vi "Configuration Tool Main.vi"() -> ()   [LabVIEW 2013, in "Advanced Configuration Tool.lvlib"]
doc: "This is the main VI for the configuration editor."
uses:
  Advanced Configuration Tool.lvlib
  Controls/StateCluster.ctl
  CEF_TreeControl/Repository/NISE_CEF_Repository.lvclass
  CEF_TreeControl/Node/NodeRef.ctl
  CEF_TreeControl/Node/NISE_CEF_Node.lvclass
  CEF_TreeControl/Node/UserEventRef.ctl
  CEF_TreeControl/Controls/EventCluster.ctl
  Controls/AddMessage.ctl
  Controls/MoveMessage.ctl
  <vilib>/Utility/error.llb/DialogType.ctl
  Classes/cRIO node/cRIO  node root.lvclass
  CEF_TreeControl/hierarchy repo/NISE_CEF_HierarchyRepo.lvclass
  <vilib>/NI/AMC/Read Termination Message.vi
  <vilib>/NI/AMC/Create Single Message.vi
  <vilib>/NI/AMC/Update Message Routing Info.vi
  <vilib>/NI/AMC/Send Message.vi
  <vilib>/NI/AMC/Globals.vi
  <vilib>/NI/AMC/AMC.lvlib
  CEF_TreeControl/NISE_CEF_TreeControl.lvlib
panel:
  in  "View":string(tree)
  in  "Exit":bool
  # "Configurator"
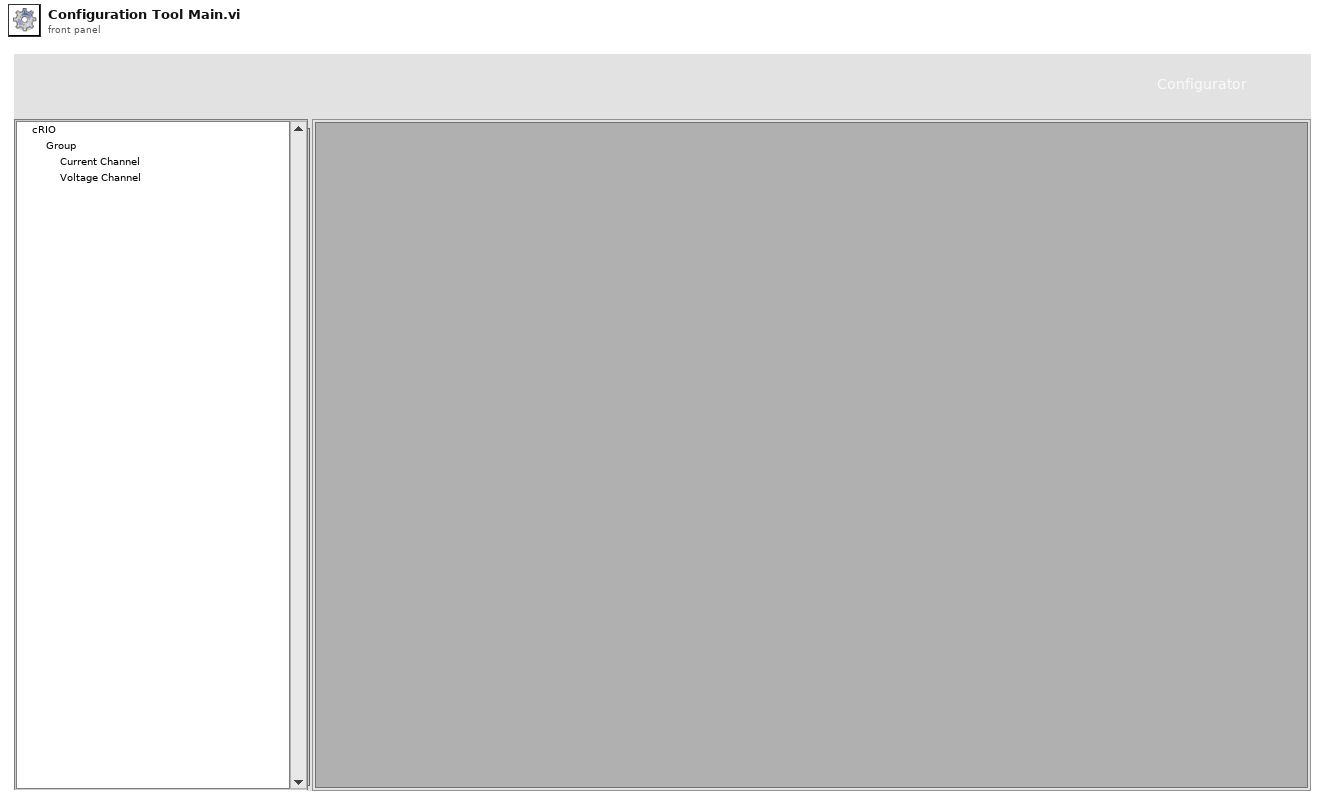
[diagram p1: front panel]
types:
  T1 = typedef "Advanced Configuration Tool.lvlib/StateCluster.ctl" = cluster{"repository":refnum<class "NISE_CEF_Repository.lvclass">, "root":T2, "unsaved changes":bool, "current path":path, "user event ref":T3, "glyph path":path, "classes path":path}
  T2 = typedef "NISE_CEF_Node.lvclass/NodeRef.ctl" = refnum<data-value>
  T3 = typedef "NISE_CEF_Node.lvclass/UserEventRef.ctl" = refnum<user-event>
  T4 = typedef "AMC.lvlib/Message Queue.ctl" = refnum<queue>
  T5 = typedef "Advanced Configuration Tool.lvlib/AddMessage.ctl" = cluster{"node type":string, "to add to":string}
  T6 = typedef "Advanced Configuration Tool.lvlib/MoveMessage.ctl" = cluster{"node ref":T2, "new parent":T2}
  T7 = typedef "NISE_CEF_TreeControl.lvlib/EventCluster.ctl" = cluster{"command":string, "data":string}
  T8 = typedef "Advanced Configuration Tool.lvlib/FilePaths.ctl" = cluster{"glyphs":path, "classes":path}
  T9 = typedef "DialogType.ctl" = u16
  T10 = typedef "NISE_CEF_Node.lvclass/Summary.ctl" = cluster{"ID":string, "parent ID":string, "node type":string, "text":string, "additional text":string, "glyph":string, "depth":i32}
  T11 = typedef "LVPoint32TypeDef.ctl" = cluster{"Horizontal":i32, "Vertical":i32}
  T12 = cluster{"data name":string, "drag data":variant}[]
  T13 = typedef "NISE_CEF_Node.lvclass/NodeMenuOptions.ctl" = cluster{"removable":bool, "movable":bool, "duplicate":bool}
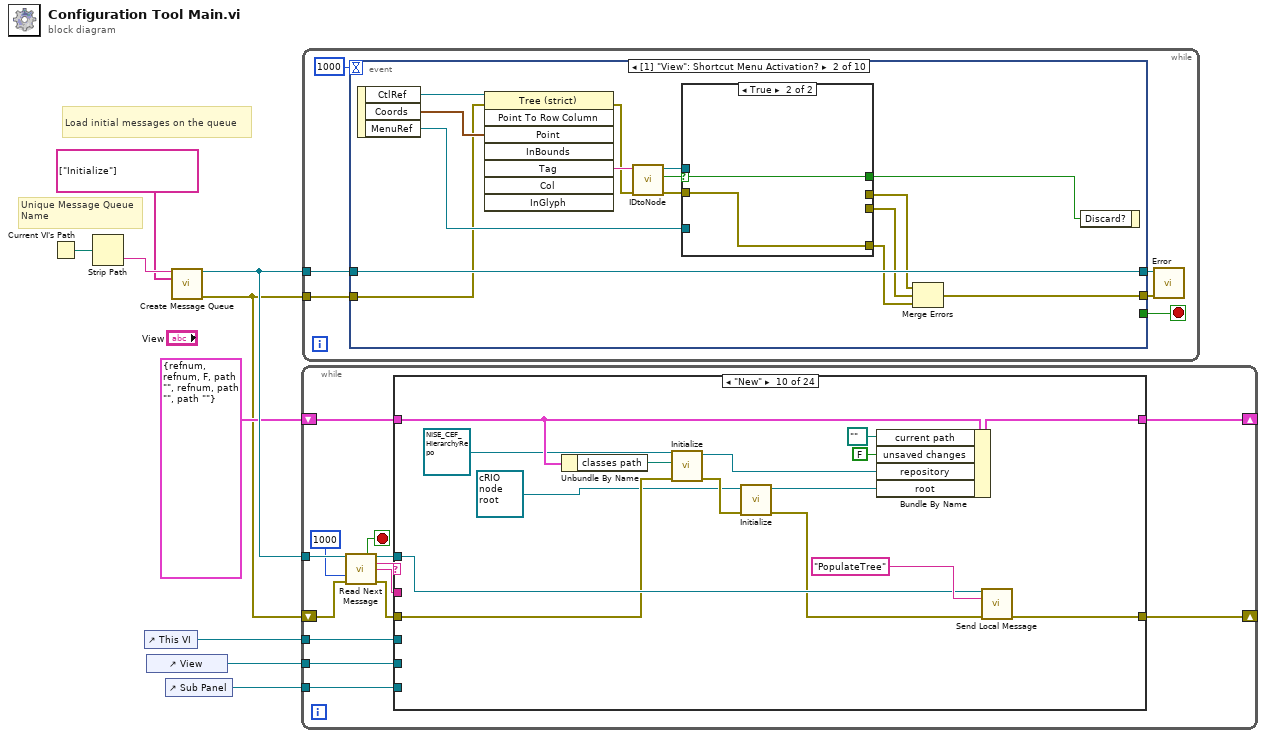
[diagram p0: block diagram]
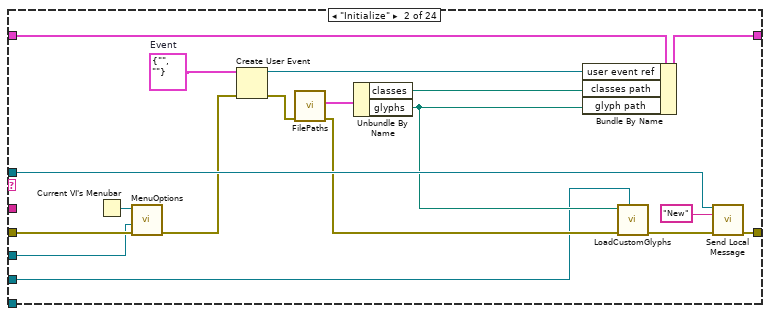
[diagram p3: hidden frame]
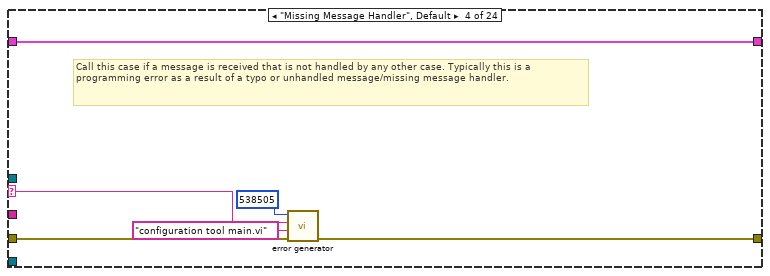
[diagram p5: hidden frame]
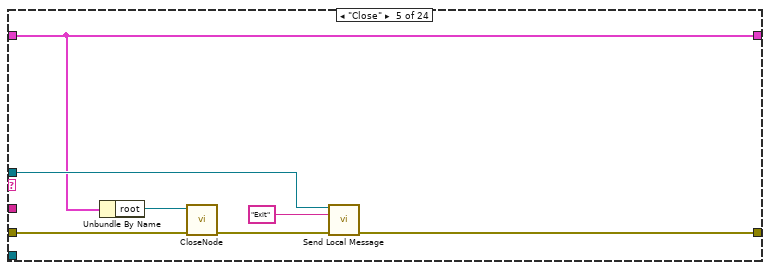
[diagram p6: hidden frame]
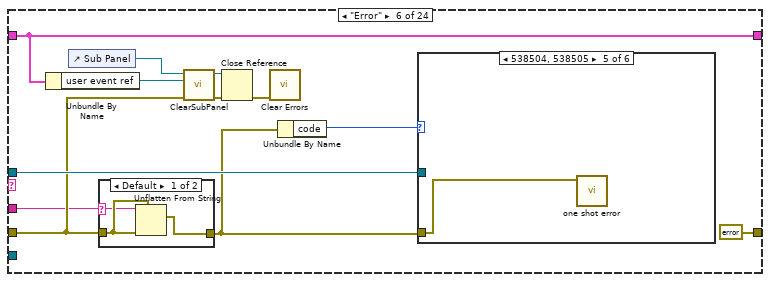
[diagram p7: hidden frame]
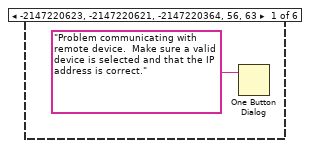
[diagram p9: hidden frame]
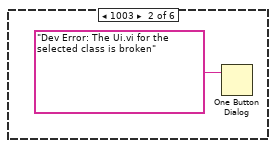
[diagram p10: hidden frame]
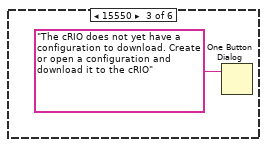
[diagram p11: hidden frame]
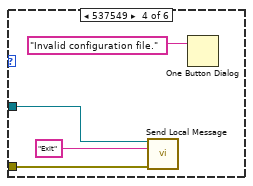
[diagram p12: hidden frame]
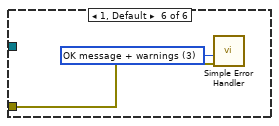
[diagram p13: hidden frame]
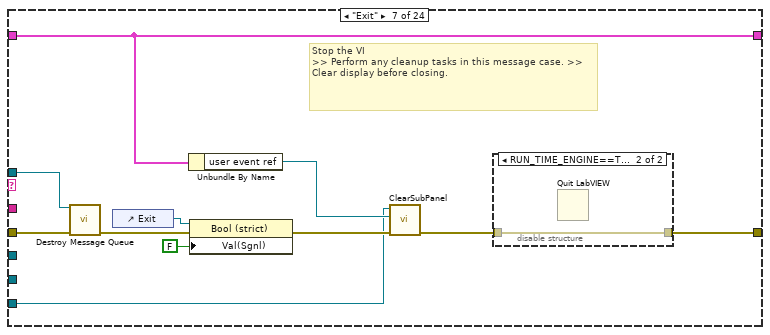
[diagram p14: hidden frame]
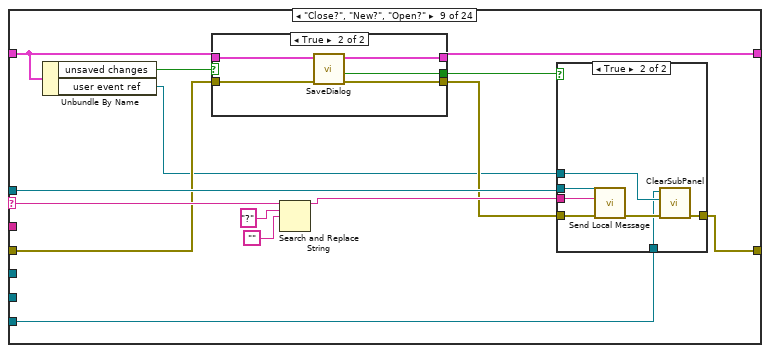
[diagram p17: hidden frame]
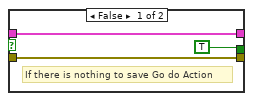
[diagram p18: hidden frame]
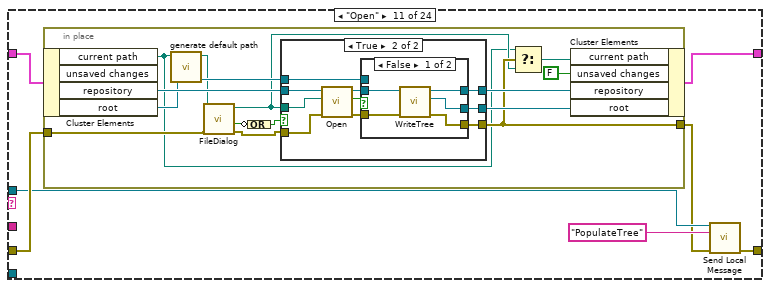
[diagram p20: hidden frame]
diagram:
  # "Unique Message Queue Name"
  # "Load initial messages on the queue"
  n1 = Current VI's Path() -> (path=w8:path)
  n2 = Strip Path(path=w8) -> (name=w9:string)  [unwired: 1 out]
  n3 = control-ref of="This VI"() -> (w3:refnum<vi>)
  n4 = control-ref of="View"() -> (w2:refnum<vi>)
  n5 = control-ref of="Sub Panel"() -> (w1:refnum<vi>)
  n6 = call <vilib>:"Create Message Queue.vi"("message queue name"=w9, "initial message names"=string[] ["Initialize"]) -> ("message queue out"=w6:T4, "error out"=w4:errorcluster)  [unwired: 12 in]
  n7 = while "Message Processor" {
    shift-right: [w19] -> _
    shift-left: w4 -> [w18]
    tunnel: w6 -> [w17]
    shift-right: [w15] -> _
    shift-left: T1 {"repository"=refnum, "root"=refnum, "unsaved changes"=FALSE, "current path"=path "", "user event ref"=refnum, "glyph path"=path "", "classes path"=path ""} -> [w14]
    tunnel: w3 -> [w12]
    tunnel: w2 -> [w11]
    tunnel: w1 -> [w10]
    stop <- w23 stop-if-true
    n8 = call <vilib>:"Read Next Message.vi"("message queue in"=w17, "timeout (1 ms)"=1000, "error in"=w18) -> ("exit process?"=w23:bool, "message queue out"=w13:T4, "message name"=w22:string, "message value"=w21:string, "error out"=w20:errorcluster)  [unwired: 5 in, 3 out]
    n9 = case shown="\"New\"" w22 {
      selector: w22 -> [_ _ _ w47 _ _ _ _ w109 _ _ _ _ _ _ _ _ w292 _ _ _ _ _ _]
      tunnel: w21 -> [_ _ _ _ _ w59 _ _ _ _ _ _ _ w223 _ w260 w272 w290 w326 w348 _ _ w391 w411]
      tunnel: w20 -> [w25 w43 w45 w50 w53 w62 w95 w99 w102 w134 w149 w189 w215 w230 w243 w250 w271 w295 w328 w347 w372 w381 w390 w409]
      tunnel: [w25 w39 w45 w48 w57 errorcluster {"status"=FALSE, "code"=0, "source"=""} ("error out") w88 w99 w113 w143 w145 w193 w217 w227 w243 w252 w275 w298 w332 w344 w367 w376 w387 w404] -> w19
      tunnel: [w24 w34 w44 w51 w55 w67 w87 w98 w104 w141 w150 w196 w216 w224 w242 w247 w276 w299 w330 w349 w374 w380 w385 w412] -> w15
      tunnel: w14 -> [w24 w35 w44 w51 w55 w67 w87 w98 w105 w138 w151 w191 w214 w225 w242 w248 w276 w299 w331 w349 w374 w380 w385 w412]
      tunnel: w13 -> [_ w38 _ _ w56 w70 w94 _ w112 w142 w147 w192 _ w226 _ _ _ w293 _ _ _ _ w386 w403]
      tunnel: w12 -> [_ w26 _ _ _ _ _ _ _ _ _ _ _ _ _ _ _ _ _ _ w359 _ _ _]
      tunnel: w11 -> [_ w27 _ _ _ _ _ _ _ _ _ _ _ _ _ w244 w269 w287 w323 w342 w360 _ _ _]
      tunnel: w10 -> [_ _ _ _ _ _ w85 _ w100 _ _ _ _ _ _ _ _ _ _ _ w357 w375 w382 _]
      frame "------------Generic Operations------------" {
        # "Dummy case to add a seperation in the Case Structure menu"
      }
      frame "Initialize" {
        w29 = T7 {"command"="", "data"=""}  # Event
        n10 = Current VI's Menubar() -> (w42:refnum<k9>)
        n11 = call "MenuOptions.vi"("error in"=w43, "VI ref"=w26, "menu ref in"=w42) -> ("error out"=w33:errorcluster)  [unwired: 7 in, 1 out]
        n12 = Create User Event(user event datatype=w29, error in=w33) -> (user event=w28:refnum<user-event>, error out=w32:errorcluster)
        n13 = call "FilePaths.vi"("error in"=w32) -> ("error out"=w37:errorcluster, "paths"=w36:T8)  [unwired: 9 in]
        n14 = Unbundle By Name(w36) -> ("classes"=w31:path, "glyphs"=w30:path)
        n15 = Bundle By Name(cluster=w35, "user event ref"=w28, "classes path"=w31, "glyph path"=w30) -> (w34:T1)
        n16 = call "LoadCustomGlyphs.vi"("tree ref"=w27, "error in"=w37, "glyph directory"=w30) -> ("error out"=w40:errorcluster)  [unwired: 8 in]
        n17 = call <vilib>:"Send Local Message.vi"("message queue in"=w38, "message name"="New" ("Message Name"), "error in"=w40) -> ("error out"=w39:errorcluster)  [unwired: 10 in, 2 out]
      }
      frame "", "Idle" {
      }
      frame "Missing Message Handler", Default {
        # "Call this case if a message is received that is not handled by any other case. Typically this is a programming error as a result of a typo or unhandled message/missing message handler."
        n18 = call "error generator.vi"("error in"=w50, "source"="configuration tool main.vi", "append error message"=w47, "error code (0)"=538505) -> ("error out"=w48:errorcluster)  [unwired: 5 in]
      }
      frame "Close" {
        n19 = Unbundle By Name(w55) -> ("root"=w54:T2)
        n20 = call "CloseNode.vi"("error in"=w53, "node ref"=w54) -> ("error out"=w52:errorcluster)  [unwired: 9 in]
        n21 = call <vilib>:"Send Local Message.vi"("message queue in"=w56, "message name"="Exit", "error in"=w52) -> ("error out"=w57:errorcluster)  [unwired: 10 in, 2 out]
      }
      frame "Error" {
        n22 = Unbundle By Name(w67) -> ("user event ref"=w65:T3)
        n23 = control-ref of="Sub Panel"() -> (w66:refnum<vi>)
        n24 = case shown="Default" w59 {
          selector: w59 -> [w72 _]
          tunnel: w62 -> [w73 w74]
          tunnel: [w71 w74] -> w61
          frame Default {
            n25 = Unflatten From String(type=w73, binary string=w72, error in (no error)=w73) -> (value=w71:errorcluster)  [unwired: 2 in, 2 out]
          }
          frame "" {
          }
        }
        n26 = call "ClearSubPanel.vi"("error in"=w62, "user event ref"=w65, "sub panel ref in"=w66) -> ("error out"=w64:errorcluster, "sub panel ref out"=w63:refnum<vi>)  [unwired: 7 in]
        n27 = Close Reference(reference=w63, error in (no error)=w64) -> (error out=w60:errorcluster)
        n28 = call <vilib>:"Clear Errors.vi"("error in (no error)"=w60) -> ()  [unwired: 6 in, 1 out]
        n29 = Unbundle By Name(w61) -> ("code"=w68:i32)
        n30 = case shown="538504, 538505" w68 {
          tunnel: w70 -> [_ _ _ w80 _ _]
          tunnel: w61 -> [_ _ _ w79 w82 w84]
          frame -2147220623, -2147220621, -2147220364, 56, 63 {
            n31 = One Button Dialog(message="Problem communicating with remote device.  Make sure a valid device is selected and that the IP address is correct.") -> ()  [unwired: 1 in, 1 out]
          }
          frame 1003 {
            n32 = One Button Dialog(message="Dev Error: The Ui.vi for the selected class is broken") -> ()  [unwired: 1 in, 1 out]
          }
          frame 15550 {
            n33 = One Button Dialog(message="The cRIO does not yet have a configuration to download. Create or open a configuration and download it to the cRIO") -> ()  [unwired: 1 in, 1 out]
          }
          frame 537549 {
            n34 = call <vilib>:"Send Local Message.vi"("message queue in"=w80, "message name"="Exit", "error in"=w79) -> ()  [unwired: 10 in, 3 out]
            n35 = One Button Dialog(message="Invalid configuration file.") -> ()  [unwired: 1 in, 1 out]
          }
          frame 538504, 538505 {
            n36 = call "one shot error.vi"("error in"=w82) -> ()  [unwired: 11 in]
          }
          frame 1, Default {
            w83 = T9 3 items=["no dialog", "OK message", "continue or stop message", "OK message + warnings", "continue/stop + warnings"] ("type of dialog (OK msg:1)")
            n37 = call <vilib>:"Simple Error Handler.vi"("type of dialog (OK msg:1)"=w83, "error in (no error)"=w84) -> ()  [unwired: 8 out]
          }
        }
      }
      frame "Exit" {
        # "Stop the VI                                                                             >> Perform any cleanup tasks in this message case. >> Clear display before closing."
        n38 = call <vilib>:"Destroy Message Queue.vi"("message queue in"=w94, "error in"=w95) -> ("error out"=w91:errorcluster)  [unwired: 11 in, 2 out]
        n39 = control-ref of="Exit"() -> (w93:refnum<vi>)
        n40 = Unbundle By Name(w87) -> ("user event ref"=w86:T3)
        n41 = property class="Bool (strict)"(reference=w93, error in=w91, "Val(Sgnl)"=FALSE ("Exit")) -> (error out=w90:errorcluster)  [unwired: 1 out]
        n42 = call "ClearSubPanel.vi"("error in"=w90, "user event ref"=w86, "sub panel ref in"=w85) -> ("error out"=w89:errorcluster)  [unwired: 7 in, 1 out]
        n43 = disable-structure shown="RUN_TIME_ENGINE==True" {
          disable-tunnel: [w96 w97] -> w88
          disable-tunnel: w89 -> [w96 w97]
          frame condition #0 (active) {
          }
          frame condition #1 {
            n44 = Quit LabVIEW() -> ()  [unwired: 1 in]
          }
        }
      }
      frame "------------Menu Operations--------------" {
        # "Dummy case to add a seperation in the Case Structure menu"
      }
      frame "Close?", "New?", "Open?" {
        n45 = Unbundle By Name(w105) -> ("unsaved changes"=w107:bool, "user event ref"=w101:T3)
        n46 = case shown="True" w107 {
          tunnel: [TRUE ("SaveFlag") w121] -> w106
          tunnel: w105 -> [w115 w120]
          tunnel: [w115 w119] -> w104
          tunnel: w102 -> [w114 w118]
          tunnel: [w114 w117] -> w103
          frame False {
            # "If there is nothing to save Go do Action"
          }
          frame True {
            n47 = call "SaveDialog.vi"("error in"=w118, "state in"=w120) -> ("error out"=w117:errorcluster, "new"=w121:bool, "state out"=w119:T1)  [unwired: 7 in]
          }
        }
        n48 = Search and Replace String(input string=w109, search string="?", replace string="") -> (result string=w108:string)  [unwired: 5 in, 3 out]
        n49 = case shown="True" w106 {
          tunnel: w103 -> [w122 w129]
          tunnel: [w122 w125] -> w113
          tunnel: w112 -> [_ w128]
          tunnel: w108 -> [_ w127]
          tunnel: w101 -> [_ w124]
          tunnel: w100 -> [_ w123]
          frame False {
          }
          frame True {
            n50 = call <vilib>:"Send Local Message.vi"("message queue in"=w128, "message name"=w127, "error in"=w129) -> ("error out"=w126:errorcluster)  [unwired: 10 in, 2 out]
            n51 = call "ClearSubPanel.vi"("error in"=w126, "user event ref"=w124, "sub panel ref in"=w123) -> ("error out"=w125:errorcluster)  [unwired: 7 in, 1 out]
          }
        }
      }
      frame "New" {
        n52 = Unbundle By Name(w138) -> ("classes path"=w137:path)
        n53 = call-dynamic "Initialize.vi"("error in"=w134, "path"=w137, "repository in"=refnum<class "NISE_CEF_HierarchyRepo.lvclass"> refnum ("NISE_CEF_HierarchyRepo.lvclass")) -> ("error out"=w136:errorcluster, "repository out"=w139:refnum<class "NISE_CEF_HierarchyRepo.lvclass">)  [unwired: 7 in]
        n54 = call-dynamic "Initialize.vi"("error in"=w136, "cRIO in"=refnum<class "cRIO  node root.lvclass"> refnum ("_cRIO.lvclass")) -> ("error out"=w135:errorcluster, "data value reference"=w140:T2)  [unwired: 7 in, 1 out]
        n55 = Bundle By Name(cluster=w138, "current path"=path "", "unsaved changes"=FALSE, "repository"=w139, "root"=w140) -> (w141:T1)
        n56 = call <vilib>:"Send Local Message.vi"("message queue in"=w142, "message name"="PopulateTree", "error in"=w135) -> ("error out"=w143:errorcluster)  [unwired: 10 in, 2 out]
      }
      frame "Open" {
        n57 = in-place {
          in-place-border: w149 -> [w157]
          in-place-border: [w156] -> w146
          n58 = in-place-cluster #1(w151) -> ("current path"=w153:path, "repository"=w165:refnum<class "NISE_CEF_Repository.lvclass">, "root"=w161:T2)  [unwired: 1 out]
          n59 = call "generate default path.vi"("current file path"=w153) -> ("browse path"=w152:path)  [unwired: 10 in]
          n60 = call "FileDialog.vi"("error in"=w157, "start path"=w152) -> ("error out"=w158:errorcluster, "cancelled"=w159:bool, "selected path"=w155:path)  [unwired: 7 in]
          n61 = Compound Arithmetic op=OR(invert w159) -> (w160:bool)
          n62 = case shown="True" w160 {
            tunnel: w165 -> [w166 w178]
            tunnel: [w166 w176] -> w163
            tunnel: [w167 w174] -> w156
            tunnel: [w168 w173] -> w162
            tunnel: w155 -> [_ w171]
            tunnel: w158 -> [w167 w170]
            tunnel: w161 -> [w168 w169]
            frame False {
            }
            frame True {
              n63 = call-dynamic "Open.vi"("error in"=w170, "file path"=w171, "repository in"=w178) -> ("error out"=w175:errorcluster, "invalid?"=w172:bool, "repository out"=w177:refnum<class "NISE_CEF_Repository.lvclass">)  [unwired: 6 in]
              n64 = case shown="False" w172 {
                tunnel: w177 -> [w183 w186]
                tunnel: [w182 w186] -> w176
                tunnel: w175 -> [w181 w185]
                tunnel: [w180 w185] -> w174
                tunnel: [w179 w184] -> w173
                tunnel: w169 -> [_ w184]
                frame False {
                  n65 = call-dynamic "WriteTree.vi"("error in"=w181, "repository in"=w183) -> ("error out"=w180:errorcluster, "root"=w179:T2, "repository out"=w182:refnum<class "NISE_CEF_Repository.lvclass">)  [unwired: 7 in]
                }
                frame True {
                }
              }
            }
          }
          n66 = Select(t=w153, s=w156, f=w155) -> (s? t:f=w154:path)
          n67 = in-place-cluster #1("current path"=w154, "unsaved changes"=FALSE ("SaveFlag"), "repository"=w163, "root"=w162) -> (w150:T1)
        }
        n68 = call <vilib>:"Send Local Message.vi"("message queue in"=w147, "message name"="PopulateTree", "error in"=w146) -> ("error out"=w145:errorcluster)  [unwired: 10 in, 2 out]
      }
      frame "Save" {
        n69 = in-place {
          in-place-border: w189 -> [w200]
          in-place-border: [w199] -> w188
          in-place-border: [w197] -> w187
          n70 = in-place-cluster #2(w191) -> ("current path"=w198:path, "root"=w201:T2, "repository"=w203:refnum<class "NISE_CEF_Repository.lvclass">)
          n71 = Empty String/Path?(string/path=w198) -> (empty?=w197:bool)
          n72 = call-dynamic "ReadTree.vi"("error in"=w200, "root"=w201, "repository in"=w203) -> ("error out"=w199:errorcluster, "repository out"=w202:refnum<class "NISE_CEF_Repository.lvclass">)  [unwired: 7 in]
          n73 = in-place-cluster #2("current path"=w198, "root"=w201, "repository"=w202) -> (w190:T1)
        }
        n74 = case shown="True" w187 {
          tunnel: w190 -> [w207 w209]
          tunnel: [w206 w208] -> w196
          tunnel: [w205 w210] -> w194
          tunnel: w188 -> [w204 w211]
          frame False {
            n75 = call "Save.vi"("error in"=w204, "state in"=w207) -> ("error out"=w205:errorcluster, "state out"=w206:T1)  [unwired: 8 in]
          }
          frame True {
            # "Empty path use Dialog"
            n76 = call "SaveAs.vi"("error in"=w211, "state in"=w209) -> ("error out"=w210:errorcluster, "state out"=w208:T1)  [unwired: 7 in, 1 out]
          }
        }
        n77 = call <vilib>:"Send Local Message.vi"("message queue in"=w192, "message name"="PopulateTree", "error in"=w194) -> ("error out"=w193:errorcluster)  [unwired: 10 in, 2 out]
      }
      frame "SaveAs" {
        n78 = in-place {
          in-place-border: w215 -> [w219]
          in-place-border: [w218] -> w213
          n79 = in-place-cluster #3(w214) -> ("root"=w220:T2, "repository"=w222:refnum<class "NISE_CEF_Repository.lvclass">)
          n80 = call-dynamic "ReadTree.vi"("error in"=w219, "root"=w220, "repository in"=w222) -> ("error out"=w218:errorcluster, "repository out"=w221:refnum<class "NISE_CEF_Repository.lvclass">)  [unwired: 7 in]
          n81 = in-place-cluster #3("root"=w220, "repository"=w221) -> (w212:T1)
        }
        n82 = call "SaveAs.vi"("error in"=w213, "state in"=w212) -> ("error out"=w217:errorcluster, "state out"=w216:T1)  [unwired: 7 in, 1 out]
      }
      frame "Custom View" {
        n83 = in-place {
          in-place-border: w230 -> [w241]
          in-place-border: [w240] -> w228
          in-place-border: w223 -> [w231]
          n84 = in-place-cluster #4(w225) -> ("repository"=w235:refnum<class "NISE_CEF_Repository.lvclass">, "root"=w234:T2)
          n85 = call-dynamic "ReadTree.vi"("error in"=w241, "root"=w234, "repository in"=w235) -> ("error out"=w238:errorcluster, "repository out"=w237:refnum<class "NISE_CEF_Repository.lvclass">)  [unwired: 7 in]
          n86 = call-dynamic "CustomView.vi"("error in"=w238, "view name"=w231, "repository in"=w237) -> ("error out"=w239:errorcluster, "repository out"=w236:refnum<class "NISE_CEF_Repository.lvclass">)  [unwired: 7 in]
          n87 = call-dynamic "WriteTree.vi"("error in"=w239, "repository in"=w236) -> ("error out"=w240:errorcluster, "root"=w232:T2, "repository out"=w233:refnum<class "NISE_CEF_Repository.lvclass">)  [unwired: 7 in]
          n88 = in-place-cluster #4("repository"=w233, "root"=w232) -> (w224:T1)
        }
        n89 = call <vilib>:"Send Local Message.vi"("message queue in"=w226, "message name"="PopulateTree", "error in"=w228) -> ("error out"=w227:errorcluster)  [unwired: 10 in, 2 out]
      }
      frame "-------TreeControl Operations-----------" {
        # "Dummy case to add a seperation in the Case Structure menu"
      }
      frame "AddNode" {
        n90 = Unflatten From String(type=T5 {"node type"="", "to add to"=""} ("input cluster"), binary string=w260) -> (value=w258:T5)  [unwired: 3 in, 2 out]
        n91 = Unbundle By Name(w258) -> ("to add to"=w255:string, "node type"=w246:string)
        n92 = in-place {
          in-place-border: w250 -> [w266]
          in-place-border: [w265] -> w249
          in-place-border: w246 -> [w264]
          in-place-border: [w263] -> w245
          n93 = in-place-cluster #5(w248) -> ("repository"=w268:refnum<class "NISE_CEF_Repository.lvclass">)
          n94 = call-dynamic "GetClassPath.vi"("error in"=w266, "class name"=w264, "Repository in"=w268) -> ("error out"=w265:errorcluster, "class path"=w263:path, "Repository out"=w267:refnum<class "NISE_CEF_Repository.lvclass">)  [unwired: 6 in]
          n95 = in-place-cluster #5("repository"=w267) -> (w247:T1)
        }
        n96 = call <vilib>:"Get LV Class Default Value.vi"("error in (no error)"=w249, "class path"=w245) -> ("error out"=w261:errorcluster, "object"=w262:refnum<class>)  [unwired: 8 in]
        n97 = To More Specific Class(target class=refnum<class "NISE_CEF_Node.lvclass"> refnum ("Node.lvclass"), reference=w262, error in=w261) -> (specific class reference=w257:refnum<class "NISE_CEF_Node.lvclass">, error out=w254:errorcluster)
        n98 = call "AddNode.vi"("error in"=w254, "node in"=w257, "parent node ID"=w255) -> ("error out"=w253:errorcluster, "summary"=w251:T10[])  [unwired: 7 in]
        n99 = call "PopulateTreeSumary.vi"("error in"=w253, "array"=w251, "tree ref in"=w244) -> ("error out"=w252:errorcluster)  [unwired: 8 in]
      }
      frame "Duplicate" {
        n100 = call "IDtoNode.vi"("error in"=w271, "ID"=w272) -> ("error out"=w273:errorcluster, "invalid Id"=w270:bool, "node ref"=w274:T2)  [unwired: 7 in]
        n101 = case shown="False" w270 {
          tunnel: [w285 w286] -> w275
          tunnel: w274 -> [w284 _]
          tunnel: w273 -> [w281 w286]
          tunnel: w269 -> [w277 _]
          frame False {
            n102 = call "DuplicateNode.vi"("same parent?"=TRUE ("s"), "error in"=w281, "node ref in"=w284) -> ("error out"=w282:errorcluster, "new node ref"=w283:T2)  [unwired: 7 in]
            n103 = call "Summary.vi"("error in"=w282, "node self ref"=w283) -> ("error out"=w279:errorcluster, "summary"=w278:T10[])  [unwired: 8 in]
            n104 = call "PopulateTreeSumary.vi"("error in"=w279, "array"=w278, "tree ref in"=w277) -> ("error out"=w285:errorcluster)  [unwired: 8 in]
          }
          frame True {
          }
        }
      }
      frame "CustomMenuAction" {
        n105 = Match Pattern(string=w290, regular expression=":") -> (before substring=w289:string, after substring=w288:string)  [unwired: 1 in, 2 out]
        n106 = call "IDtoNode.vi"("error in"=w295, "ID"=w288) -> ("error out"=w296:errorcluster, "invalid Id"=w294:bool, "node ref"=w297:T2)  [unwired: 7 in]
        n107 = case shown="False" w294 {
          tunnel: [w302 w322] -> w298
          tunnel: w297 -> [w307 _]
          tunnel: w296 -> [w305 w322]
          tunnel: w293 -> [w306 _]
          tunnel: w292 -> [_ _]
          tunnel: w289 -> [w303 _]
          tunnel: w287 -> [w300 _]
          frame False {
            n108 = in-place {
              in-place-border: w306 -> [w320]
              in-place-border: w305 -> [w318]
              in-place-border: [w317] -> w301
              in-place-border: [w316] -> w304
              in-place-border: w303 -> [w315]
              in-place-border: w300 -> [w314]
              n109 = in-place-dvr #6(w307) -> (w321:refnum<class "NISE_CEF_Node.lvclass">)  [unwired: 1 out]
              n110 = call-dynamic "MenuHandler.vi"("tree control"=w314, "message queue out"=w320, "error in (no error)"=w318, "menu string"=w315, "NISE_CEF_Node in"=w321) -> ("error out"=w317:errorcluster, "Unhandled"=w316:bool, "NISE_CEF_Node out"=w319:refnum<class "NISE_CEF_Node.lvclass">)  [unwired: 4 in]
              n111 = in-place-dvr #6(w319) -> ()  [unwired: 2 out]
            }
            n112 = case shown="True" w304 {
              tunnel: w303 -> [_ w309]
              tunnel: [w308 w310] -> w302
              tunnel: w301 -> [w308 w311]
              frame False {
              }
              frame True {
                n113 = call "error generator.vi"("error in"=w311, "source"="configuration tool main.vi", "append error message"=w309, "error code (0)"=538506) -> ("error out"=w310:errorcluster)  [unwired: 5 in]
              }
            }
          }
          frame True {
          }
        }
      }
      frame "RefreshNode" {
        # "Refreshes the node in the Tree               Sets the save flag to true                       This case can be called from the UIs of the nodes"
        n114 = call "IDtoNode.vi"("error in"=w328, "ID"=w326) -> ("error out"=w327:errorcluster, "invalid Id"=w324:bool, "node ref"=w325:T2)  [unwired: 7 in]
        n115 = case shown="False" w324 {
          tunnel: [w339 w341] -> w332
          tunnel: w327 -> [w335 w341]
          tunnel: w325 -> [w334 _]
          tunnel: w323 -> [w333 _]
          frame False {
            n116 = call "Summary.vi"("error in"=w335, "node self ref"=w334) -> ("error out"=w337:errorcluster, "summary"=w336:T10[])  [unwired: 8 in]
            n117 = call "RefreshSubTree.vi"("error in"=w337, "node information"=w336, "tree ref in"=w333) -> ("error out"=w340:errorcluster, "tree ref out"=w338:refnum<vi>)  [unwired: 7 in]
            n118 = Close Reference(reference=w338, error in (no error)=w340) -> (error out=w339:errorcluster)
          }
          frame True {
          }
        }
        n119 = Bundle By Name(cluster=w331, "unsaved changes"=TRUE ("SaveFlag")) -> (w330:T1)
      }
      frame "RemoveNode" {
        n120 = call "IDtoNode.vi"("error in"=w347, "ID"=w348) -> ("error out"=w346:errorcluster, "invalid Id"=w343:bool, "node ref"=w345:T2)  [unwired: 7 in]
        n121 = case shown="False" w343 {
          tunnel: w346 -> [w355 w356]
          tunnel: w345 -> [w354 _]
          tunnel: [w351 w356] -> w344
          tunnel: w342 -> [w350 _]
          frame False {
            n122 = call "RemoveNode.vi"("error in"=w355, "node"=w354) -> ("error out"=w352:errorcluster, "node ID"=w353:string)  [unwired: 8 in]
            n123 = call "ClearTreeNode.vi"("error in"=w352, "tag"=w353, "tree reference"=w350) -> ("error out"=w351:errorcluster)  [unwired: 8 in]
          }
          frame True {
          }
        }
      }
      frame "PopulateTree" {
        n124 = Unbundle By Name(w374) -> ("current path"=w365:path, "user event ref"=w366:T3, "root"=w370:T2)
        n125 = call "Summary.vi"("error in"=w372, "depth"=0 ("Depth"), "node self ref"=w370) -> ("error out"=w371:errorcluster, "summary"=w373:T10[])  [unwired: 7 in]
        n126 = call <vilib>:"Check if File or Folder Exists.vi"("path"=w365) -> ("file or folder exists?"=w363:bool, "dup path"=w364:path)  [unwired: 8 in, 1 out]
        n127 = Strip Path(path=w364) -> (name=w362:string)  [unwired: 1 out]
        n128 = call "RefreshEntireTree.vi"("calling VI in"=w359, "error in"=w371, "array"=w373, "tree ref in"=w360) -> ("error out"=w368:errorcluster)  [unwired: 7 in]
        n129 = Select(t=w362, s=w363, f="Advanced Configurator Sample Project") -> (s? t:f=w358:string)
        n130 = property class="VI"(reference=w359, "Front Panel.Title"=w358) -> ()  [unwired: 1 in, 2 out]
        n131 = call "ClearSubPanel.vi"("error in"=w368, "user event ref"=w366, "sub panel ref in"=w357) -> ("error out"=w367:errorcluster)  [unwired: 7 in, 1 out]
      }
      frame "CleansubPanel" {
        n132 = Unbundle By Name(w380) -> ("user event ref"=w379:T3)
        n133 = call "ClearSubPanel.vi"("error in"=w381, "user event ref"=w379, "sub panel ref in"=w375) -> ("error out"=w378:errorcluster, "sub panel ref out"=w377:refnum<vi>)  [unwired: 7 in]
        n134 = Close Reference(reference=w377, error in (no error)=w378) -> (error out=w376:errorcluster)
      }
      frame "ActivateNode" {
        n135 = Unbundle By Name(w385) -> ("user event ref"=w384:T3)
        n136 = call "IDtoNode.vi"("error in"=w390, "ID"=w391) -> ("error out"=w383:errorcluster, "invalid Id"=w389:bool, "node ref"=w388:T2)  [unwired: 7 in]
        n137 = case shown="True" w389 {
          tunnel: w388 -> [w398 _]
          tunnel: [w399 w400] -> w387
          tunnel: w383 -> [w396 w400]
          tunnel: w386 -> [w394 _]
          tunnel: w384 -> [w395 _]
          tunnel: w382 -> [w392 _]
          frame False {
            n138 = call "ClearSubPanel.vi"("error in"=w396, "user event ref"=w395, "sub panel ref in"=w392) -> ("error out"=w397:errorcluster, "sub panel ref out"=w393:refnum<vi>)  [unwired: 7 in]
            n139 = call "LoadNodeUI.vi"("user event out"=w395, "error in"=w397, "sub panel ref in"=w393, "main queue"=w394, "node"=w398) -> ("error out"=w399:errorcluster)  [unwired: 6 in]
          }
          frame True {
          }
        }
      }
      frame "Move" {
        n140 = Unflatten From String(type=T6 {"node ref"=refnum, "new parent"=refnum} ("Cluster"), binary string=w411, error in (no error)=w409) -> (value=w408:T6, error out=w407:errorcluster)  [unwired: 2 in, 1 out]
        n141 = Unbundle By Name(w408) -> ("node ref"=w402:T2, "new parent"=w401:T2)
        n142 = call "MoveNode.vi"("error in"=w407, "new parent"=w401, "node"=w402) -> ("error out"=w405:errorcluster)  [unwired: 8 in]
        n143 = call <vilib>:"Send Local Message.vi"("message queue in"=w403, "message name"="PopulateTree", "error in"=w405) -> ("error out"=w404:errorcluster)  [unwired: 10 in, 2 out]
      }
    }
  }
  n144 = while "User Interface Event Handler" {
    tunnel: w6 -> [w417]
    tunnel: w4 -> [w413]
    stop <- w416 stop-if-true
    n145 = event shown="[1] \"View\": Shortcut Menu Activation?" {
      selector: _ -> [_ _ _ _ _ _ _ _ _ _]
      dyn-events: _ -> [_ _ _ _ _ _ _ _ _ _]
      timeout: 1000 -> [_ _ _ _ _ _ _ _ _ _]
      tunnel: w417 -> [w420 w429 w454 w506 w534 w541 w570 w574 w584 w590]
      tunnel: [_ _ _ _ TRUE _ _ _ _ _] -> w416
      tunnel: [w420 w429 w451 w504 w530 w541 w567 w574 w582 w589] -> w415
      tunnel: [w419 w425 w450 w503 w531 w537 w566 w571 w580 w587] -> w414
      tunnel: w413 -> [w419 w428 w449 w505 w532 w540 w565 w573 w581 w588]
      event Timeout {
        # "Timeout code can be added here for autosave or Lock Screen"
        n146 = event-data() -> ()  [unwired: 1 in, 1 out]
      }
      event "View": Shortcut Menu Activation? {
        n147 = event-data() -> ("CtlRef"=w435:refnum<vi>, "Coords"=w434:T11, "MenuRef"=w431:refnum<k9>)  [unwired: 1 in]
        n148 = invoke class="Tree (strict)" method="Point To Row Column"(reference=w435, error in=w428, "Point"=w434) -> (error out=w427:errorcluster, "Tag"=w433:string)  [unwired: 5 in, 6 out]
        n149 = call "IDtoNode.vi"("error in"=w427, "ID"=w433) -> ("error out"=w423:errorcluster, "invalid Id"=w430:bool, "node ref"=w432:T2)  [unwired: 7 in]
        n150 = case shown="True" w430 {
          selector: w430 -> [_ w446]
          tunnel: w432 -> [w440 _]
          tunnel: w431 -> [w439 _]
          tunnel: [w438 _] -> w426
          tunnel: [w437 _] -> w424
          tunnel: w423 -> [w436 w447]
          tunnel: [w436 w447] -> w422
          tunnel: [_ w446] -> w421
          frame False {
            n151 = in-place {
              in-place-border: w439 -> [w443]
              in-place-border: [w441] -> w438
              n152 = in-place-dvr #7(w440) -> (w445:refnum<class "NISE_CEF_Node.lvclass">, w442:errorcluster)
              n153 = call-dynamic "ShortcutMenu.vi"("error in"=w442, "menu ref in"=w443, "node in"=w445) -> ("error out"=w441:errorcluster, "node out"=w444:refnum<class "NISE_CEF_Node.lvclass">)  [unwired: 6 in, 1 out]
              n154 = in-place-dvr #7(w444) -> (w437:errorcluster)  [unwired: 1 out]
            }
          }
          frame True {
          }
        }
        n155 = Merge Errors(w424, w426, w422) -> (w425:errorcluster)
        n156 = event-data("Discard?"=w421) -> ()  [unwired: 1 in, 1 out]
      }
      event "View": Shortcut Menu Selection (User) {
        n157 = event-data() -> ("ItemPath"=w453:string, "CtlRef"=w457:refnum<vi>, "Coords"=w458:T11)  [unwired: 1 in]
        n158 = invoke class="Tree (strict)" method="Point To Row Column"(reference=w457, error in=w449, "Point"=w458) -> (error out=w448:errorcluster, "Tag"=w452:string)  [unwired: 5 in, 6 out]
        n159 = Match Pattern(string=w453, regular expression=":") -> (before substring=w456:string, after substring=w455:string)  [unwired: 1 in, 2 out]
        n160 = case shown="Default" w456 {
          selector: w456 -> [w460 _ _ _]
          tunnel: w455 -> [_ _ _ w485]
          tunnel: w454 -> [w467 w474 w480 w487]
          tunnel: w452 -> [w462 w472 w478 w486]
          tunnel: [w464 w471 w477 w483] -> w451
          tunnel: [w465 w470 w475 w481] -> w450
          tunnel: w448 -> [w466 w469 w476 w482]
          frame Default {
            n161 = Concatenate Strings(w460, ":" ("string"), w462) -> (w463:string)
            n162 = call <vilib>:"Send Local Message.vi"("message queue in"=w467, "message name"="CustomMenuAction" ("Message Name"), "message value"=w463, "error in"=w466) -> ("message queue out"=w464:T4, "error out"=w465:errorcluster)  [unwired: 9 in, 1 out]
          }
          frame "Remove" {
            n163 = call <vilib>:"Send Local Message.vi"("message queue in"=w474, "message name"="RemoveNode" ("Message Name"), "message value"=w472, "error in"=w469) -> ("message queue out"=w471:T4, "error out"=w470:errorcluster)  [unwired: 9 in, 1 out]
          }
          frame "Duplicate" {
            n164 = call <vilib>:"Send Local Message.vi"("message queue in"=w480, "message name"="Duplicate" ("Message Name"), "message value"=w478, "error in"=w476) -> ("message queue out"=w477:T4, "error out"=w475:errorcluster)  [unwired: 9 in, 1 out]
          }
          frame "Add" {
            n165 = Bundle By Name(cluster=T5 {"node type"="", "to add to"=""} ("input cluster"), "node type"=w485, "to add to"=w486) -> (w488:T5)
            n166 = Flatten To String(anything=w488) -> (data string=w489:string)  [unwired: 3 in, 2 out]
            n167 = call <vilib>:"Send Local Message.vi"("message queue in"=w487, "message name"="AddNode" ("Message Name"), "message value"=w489, "error in"=w482) -> ("message queue out"=w483:T4, "error out"=w481:errorcluster)  [unwired: 9 in, 1 out]
          }
        }
      }
      event "View": Drop {
        n168 = event-data() -> ("CtlRef"=w509:refnum<vi>, "Coords"=w508:T11)  [unwired: 1 in]
        n169 = invoke class="Tree (strict)" method="Point To Row Column"(reference=w509, error in=w505, "Point"=w508) -> (reference out=w507:refnum<vi>, error out=w502:errorcluster, "Tag"=w499:string)  [unwired: 5 in, 5 out]
        n170 = call "ValidDragDrop.vi"("error in"=w502, "drag over"=w499, "tree ref in"=w507) -> ("error out"=w494:errorcluster, "accepted"=w497:bool, "drag"=w501:string, "tree ref out"=w511:refnum<vi>)  [unwired: 5 in]
        n171 = call "IDtoNode.vi"("error in"=w494, "ID"=w499) -> ("error out"=w495:errorcluster, "invalid Id"=w492:bool, "node ref"=w498:T2)  [unwired: 7 in]
        n172 = call "IDtoNode.vi"("error in"=w495, "ID"=w501) -> ("error out"=w493:errorcluster, "invalid Id"=w491:bool, "node ref"=w500:T2)  [unwired: 7 in]
        n173 = Compound Arithmetic op=AND(w497, invert w492, invert w491) -> (w496:bool)
        n174 = case shown="True" w496 {
          tunnel: w501 -> [_ w527]
          tunnel: w511 -> [_ w529]
          tunnel: [_ TRUE] -> w510
          tunnel: w499 -> [_ w525]
          tunnel: w506 -> [w513 w524]
          tunnel: [w513 w520] -> w504
          tunnel: [w512 w519] -> w503
          tunnel: w500 -> [_ w515]
          tunnel: w498 -> [_ w514]
          tunnel: w493 -> [w512 w516]
          frame False {
          }
          frame True {
            n175 = invoke class="Tree (strict)" method="Edit Tree Items.Move Item"(reference=w529, error in=w516, "tag"=w527, "New Parent"=w525) -> (error out=w517:errorcluster)  [unwired: 3 in, 6 out]
            n176 = Bundle By Name(cluster=T6 {"node ref"=refnum, "new parent"=refnum} ("Cluster"), "new parent"=w514, "node ref"=w515) -> (w523:T6)
            n177 = Flatten To String(anything=w523, error in (no error)=w517) -> (data string=w522:string, error out=w518:errorcluster)  [unwired: 2 in, 1 out]
            n178 = call <vilib>:"Send Local Message.vi"("message queue in"=w524, "message name"="Move", "message value"=w522, "error in"=w518) -> ("message queue out"=w520:T4, "error out"=w519:errorcluster)  [unwired: 9 in, 1 out]
          }
        }
        n179 = event-data("Accepted?"=w510) -> ()  [unwired: 1 in, 1 out]
      }
      event "Exit": Value Change {
        # "Exit the application                                           >> Stop this message generator loop    Cleaning errors if the other loop stop this one"
        n180 = event-data() -> ()  [unwired: 1 in, 1 out]
        n181 = call <vilib>:"Send Local Message.vi"("message queue in"=w534, "message name"="Close", "error in"=w532) -> ("message queue out"=w530:T4, "error out"=w535:errorcluster)  [unwired: 10 in, 1 out]
        n182 = call <vilib>:"Clear Errors.vi"("error in (no error)"=w535) -> ("error out"=w531:errorcluster)  [unwired: 6 in]
      }
      event "View": Drag Starting? {
        n183 = event-data() -> ("Data"=w547:T12, "CtlRef"=w549:refnum<vi>, "Coords"=w548:T11)  [unwired: 1 in]
        n184 = invoke class="Tree (strict)" method="Point To Row Column"(reference=w549, error in=w540, "Point"=w548) -> (error out=w539:errorcluster, "Tag"=w546:string)  [unwired: 5 in, 6 out]
        n185 = call "IDtoNode.vi"("error in"=w539, "ID"=w546) -> ("error out"=w538:errorcluster, "invalid Id"=w545:bool, "node ref"=w544:T2)  [unwired: 7 in]
        n186 = case shown="False" w545 {
          tunnel: w544 -> [w557 _]
          tunnel: [w554 TRUE ("Removable")] -> w542
          tunnel: w538 -> [w553 w563]
          tunnel: [w550 w563] -> w537
          frame False {
            n187 = in-place {
              in-place-border: [w560] -> w556
              in-place-border: w553 -> [w559]
              in-place-border: [w558] -> w552
              n188 = in-place-dvr #8(w557) -> (w562:refnum<class "NISE_CEF_Node.lvclass">)  [unwired: 1 out]
              n189 = call-dynamic "EditOptions.vi"("error in"=w559, "node in"=w562) -> ("error out"=w558:errorcluster, "edit options"=w560:T13, "node out"=w561:refnum<class "NISE_CEF_Node.lvclass">)  [unwired: 6 in, 1 out]
              n190 = in-place-dvr #8(w561) -> (w551:errorcluster)  [unwired: 1 out]
            }
            n191 = Unbundle By Name(w556) -> ("movable"=w555:bool)
            n192 = Merge Errors(w551, w552) -> (w550:errorcluster)
            n193 = Not(x=w555) -> (.not. x?=w554:bool)
          }
          frame True {
          }
        }
        n194 = event-data("Data"=w547, "Drag Mode"=enum32{"copy or move", "copy only", "move only"}."move only", "Discard?"=w542) -> ()  [unwired: 1 in, 1 out]
      }
      event "View": Value Change {
        n195 = event-data() -> ("NewVal"=w568:string)  [unwired: 1 in]
        n196 = call <vilib>:"Send Local Message.vi"("message queue in"=w570, "message name"="ActivateNode" ("Message Name"), "message value"=w568, "error in"=w565) -> ("message queue out"=w567:T4, "error out"=w566:errorcluster)  [unwired: 9 in, 1 out]
      }
      event "View": event type 3.0.xa000003a {
        n197 = event-data() -> ("CtlRef"=w579:refnum<vi>, "Coords"=w576:T11)  [unwired: 1 in]
        n198 = invoke class="Tree (strict)" method="Point To Row Column"(reference=w579, error in=w573, "Point"=w576) -> (reference out=w578:refnum<vi>, error out=w572:errorcluster, "Tag"=w577:string)  [unwired: 5 in, 5 out]
        n199 = call "ValidDragDrop.vi"("error in"=w572, "drag over"=w577, "tree ref in"=w578) -> ("error out"=w571:errorcluster, "accepted"=w575:bool)  [unwired: 5 in, 2 out]
        n200 = event-data("Accepted?"=w575) -> ()  [unwired: 1 in, 1 out]
      }
      event Panel Close? {
        # "Intercepts the upper right close panel operation to allow a smooth shutdown as opposed to immediately killing the app."
        n201 = event-data() -> ()  [unwired: 1 in, 1 out]
        n202 = call <vilib>:"Send Local Message.vi"("message queue in"=w584, "message name"="Close?", "error in"=w581) -> ("message queue out"=w582:T4, "error out"=w580:errorcluster)  [unwired: 10 in, 1 out]
        n203 = event-data("Discard?"=TRUE) -> ()  [unwired: 1 in, 1 out]
      }
      event Menu Selection (User) {
        # "#USERCFG It is needed to add a Case for Every item on the menu"
        n204 = event-data() -> ("ItemTag"=w586:string, "ItemPath"=w591:string)  [unwired: 1 in]
        n205 = case shown="Default" w591 {
          selector: w591 -> [w595 _ _ _ _ _ _]
          tunnel: w590 -> [w600 w605 w610 w615 w620 w625 w634]
          tunnel: [w600 w601 w606 w611 w616 w621 w631] -> w589
          tunnel: w588 -> [w597 w603 w608 w613 w618 w623 w630]
          tunnel: [w596 w602 w607 w612 w617 w622 w628] -> w587
          tunnel: w586 -> [w594 _ _ _ _ _ _]
          frame Default {
            n206 = Concatenate Strings(w594, "::" ("string"), w595) -> (w593:string)
            n207 = call "error generator.vi"("error in"=w597, "source"="configuration tool main.vi", "append error message"=w593, "error code (0)"=538506) -> ("error out"=w596:errorcluster)  [unwired: 5 in]
          }
          frame "_File:_New" {
            n208 = call <vilib>:"Send Local Message.vi"("message queue in"=w605, "message name"="New?" ("Message Name"), "error in"=w603) -> ("message queue out"=w601:T4, "error out"=w602:errorcluster)  [unwired: 10 in, 1 out]
          }
          frame "_File:_Open" {
            n209 = call <vilib>:"Send Local Message.vi"("message queue in"=w610, "message name"="Open?" ("Message Name"), "error in"=w608) -> ("message queue out"=w606:T4, "error out"=w607:errorcluster)  [unwired: 10 in, 1 out]
          }
          frame "_File:_Save" {
            n210 = call <vilib>:"Send Local Message.vi"("message queue in"=w615, "message name"="Save" ("Message Name"), "error in"=w613) -> ("message queue out"=w611:T4, "error out"=w612:errorcluster)  [unwired: 10 in, 1 out]
          }
          frame "_File:Save As..." {
            n211 = call <vilib>:"Send Local Message.vi"("message queue in"=w620, "message name"="SaveAs" ("Message Name"), "error in"=w618) -> ("message queue out"=w616:T4, "error out"=w617:errorcluster)  [unwired: 10 in, 1 out]
          }
          frame "_File:_Exit" {
            n212 = call <vilib>:"Send Local Message.vi"("message queue in"=w625, "message name"="Close?" ("Message Name"), "error in"=w623) -> ("message queue out"=w621:T4, "error out"=w622:errorcluster)  [unwired: 10 in, 1 out]
          }
          frame "_Tools:Multiple Parameter Editor" {
            n213 = call <vilib>:"Send Local Message.vi"("message queue in"=w634, "message name"="CleansubPanel", "error in"=w630) -> ("message queue out"=w633:T4, "error out"=w629:errorcluster)  [unwired: 10 in, 1 out]
            n214 = call <vilib>:"Send Local Message.vi"("message queue in"=w633, "message name"="Custom View" ("Message Name"), "message value"="Multiple Variable Editor" ("Message Name"), "error in"=w629) -> ("message queue out"=w631:T4, "error out"=w628:errorcluster)  [unwired: 9 in, 1 out]
          }
        }
      }
    }
    n215 = call "Error.vi"("error in (no error)"=w414, "message queue in"=w415) -> ()  [unwired: 9 in, 1 out]
  }
